vi "event_water.vi"(8 "error in":errorcluster, 9 "reference cluster in":T1, 11 "water on?":bool) -> (0 "error out":errorcluster)   [LabVIEW 2016]
uses:
  Type Definitions/reference_cluster.ctl
  Type Definitions/vars_settings.ctl
  Type Definitions/stim_type.ctl
  Type Definitions/backlight_type.ctl
  Type Definitions/vars_runtime.ctl
  Type Definitions/data.ctl
  Type Definitions/notifier_elements_GUI.ctl
  Type Definitions/notifier_elements_DAQ.ctl
  Type Definitions/notifier_elements_write.ctl
  Type Definitions/control_references.ctl
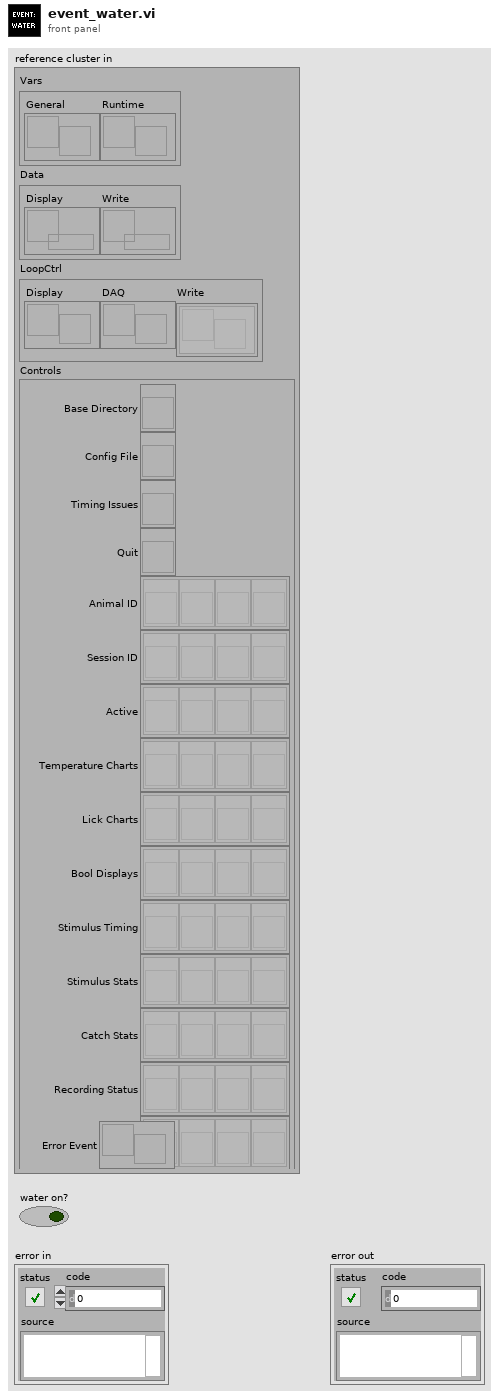
[diagram p1: front panel]
types:
  T1 = typedef "reference_cluster.ctl" = cluster{"Vars":cluster{"General":refnum<notifier>, "Runtime":refnum<notifier>}, "Data":cluster{"Display":refnum<queue>, "Write":refnum<queue>}, "LoopCtrl":cluster{"Display":refnum<notifier>, "DAQ":refnum<notifier>, "Write":refnum<notifier>[]}, "Controls":T2, "Error Event":refnum<user-event>}
  T2 = typedef "control_references.ctl" = cluster{"Base Directory":refnum<vi>, "Config File":refnum<vi>, "Timing Issues":refnum<vi>, "Quit":refnum<vi>, "Animal ID":refnum<vi>[], "Session ID":refnum<vi>[], "Active":refnum<vi>[], "Temperature Charts":refnum<vi>[], "Lick Charts":refnum<vi>[], "Bool Displays":refnum<vi>[], "Stimulus Timing":refnum<vi>[], "Stimulus Stats":refnum<vi>[], "Catch Stats":refnum<vi>[], "Recording Status":refnum<vi>[], "Pairing":refnum<vi>[]}
  T3 = typedef "vars_settings.ctl" = cluster{"base directory":path, "data directory":path, "active":bool, "running":bool, "pairing":bool, "clean tubes":bool, "animal ID":u16, "session ID":u16, "base temp":dbl, "d wait min":u16, "d wait max":u16, "d timeout":u16, "d timeout catch":u16, "d reward":u16, "n reward":u16, "idx stim":u16, "timeout win":u16, "lick win":i32[], "stim type":T4[], "stim dur":u16[], "stim amp":dbl[], "stim freq":u16[], "stim ramp":u16[], "stim catch":u8[], "pairing delay":i16[], "square dur":u16[], "square delay":i16[], "square freq":u8[], "square dc":u8[], "stim shape":dbl[][], "square shape":bool[][], "backlight type":T5, "backlight freq":u16, "dStimOne dur":u16[], "dStimOne delay":i16[], "dStimTwo dur":u16[], "dStimTwo delay":i16[]}
  T4 = typedef "stim_type.ctl" = enum16{"pulse", "vibration", "square", "sine"}
  T5 = typedef "backlight_type.ctl" = enum16{"none", "random", "regular"}
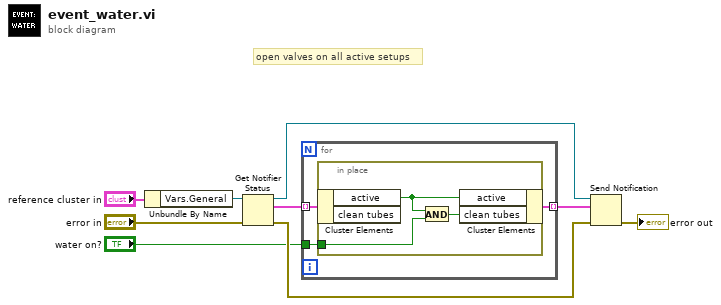
[diagram p0: block diagram]
diagram:
  # "open valves on all active setups"
  n1 = Unbundle By Name("reference cluster in") -> ("Vars.General"=w9:refnum<notifier>)
  n2 = Get Notifier Status(notifier=w9, error in (no error)="error in") -> (notifier out=w3:refnum<notifier>, current notification=w1:T3[], error out=w7:errorcluster)  [unwired: 2 out]
  n3 = for {
    tunnel: w1 -> [w12] mode=indexing
    tunnel: [w11] -> w2 mode=indexing
    tunnel: "water on?" -> [w10]
    n4 = in-place {
      in-place-border: w10 -> [w14]
      n5 = in-place-cluster #1(w12) -> ("active"=w13:bool)  [unwired: 1 out]
      n6 = And(x=w13, y=w14) -> (x .and. y?=w15:bool)
      n7 = in-place-cluster #1("active"=w13, "clean tubes"=w15) -> (w11:T3)
    }
  }
  n8 = Send Notification(notification=w2, notifier=w3, error in (no error)=w7) -> (error out=→"error out":errorcluster)  [unwired: 1 out]
